vi "Write data to PXImc.vi"(8 "error in (no error)":errorcluster, 11 "RT Data Cluster in":T1 {"StatusRefs" format="%.0x"; "ReceiveRefs"."Data Reference" format="%.0x"; "SendRefs"."Data Reference" format="%.0x"}) -> (0 "error out":errorcluster, 3 "RT Data Cluster out":T1 {"StatusRefs" format="%.0x"; "ReceiveRefs"."Data Reference" format="%.0x"; "SendRefs"."Data Reference" format="%.0x"})   [LabVIEW 2012, in "PXImc Engine.lvlib"]
uses:
  PXImc Engine.lvlib
  RT Data Cluster.ctl
  Shared/Compiled Data.ctl
  <vilib>/NI Veristand/Custom Device API/Block Data Reference.ctl
  <vilib>/NI Veristand/Custom Device API/Data Reference.ctl
  <vilib>/NI Veristand/Custom Device API/Global Data Refs.vi
  <vilib>/pximc/Write (DBL).vi
  <vilib>/pximc/nipximc.lvlib
  <vilib>/NI Veristand/Custom Device API/Custom Device API.lvlib
  <resource>/objmgr/pximc.rc
  Shared/PXImc Shared.lvlib
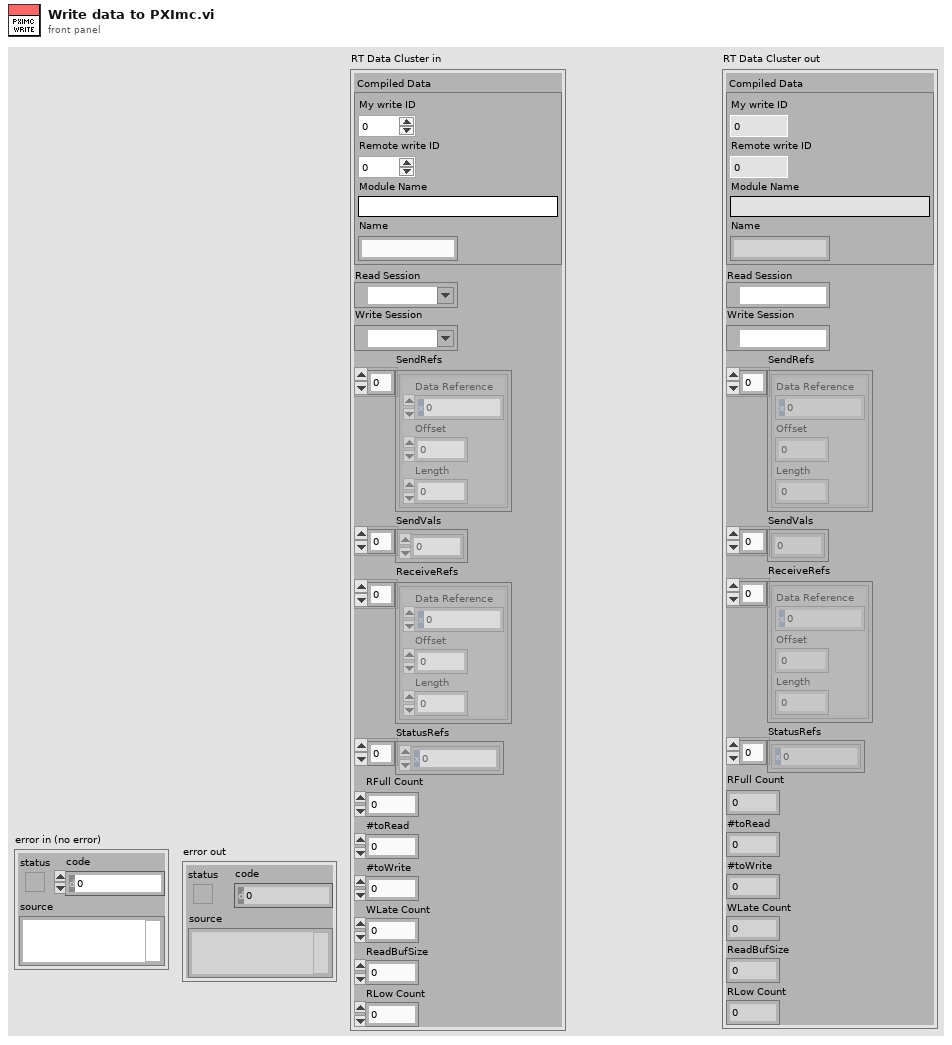
[diagram p1: front panel]
types:
  T1 = typedef "PXImc Engine.lvlib/RT Data Cluster.ctl" = cluster{"Compiled Data":T2, "Read Session":refnum<k21>, "Write Session":refnum<k21>, "SendRefs":T3[], "SendVals":dbl[], "ReceiveRefs":T3[], "StatusRefs":T4[], "RFull Count":dbl, "#toRead":i32, "#toWrite":i32, "WLate Count":dbl, "ReadBufSize":i32, "RLow Count":dbl}
  T2 = typedef "PXImc Shared.lvlib/Compiled Data.ctl" = cluster{"My write ID":u16, "Remote write ID":u16, "Module Name":string, "Name":string}
  T3 = typedef "Custom Device API.lvlib/Block Data Reference.ctl" = cluster{"Data Reference":T4, "Offset":i32, "Length":i32}
  T4 = typedef "Custom Device API.lvlib/Data Reference.ctl" = i32
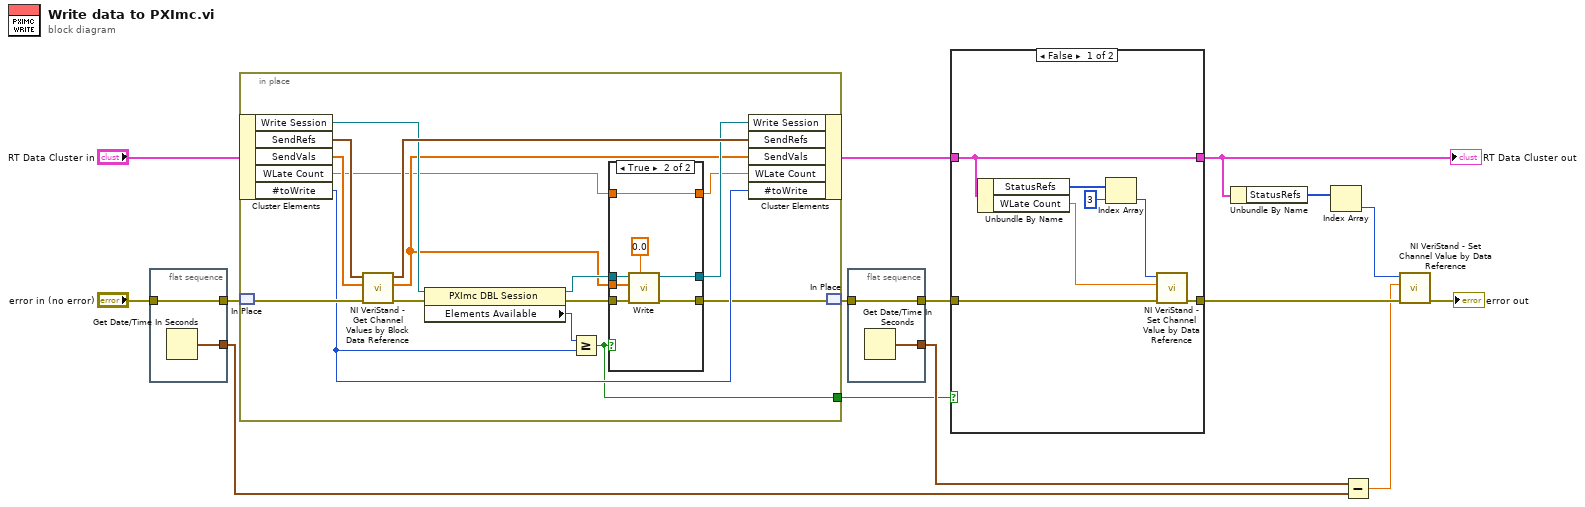
[diagram p0: block diagram]
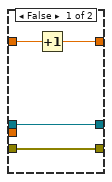
[diagram p3: hidden frame]
diagram:
  n1 = flat-sequence {
    tunnel: [w17] -> w15
    tunnel: "error in (no error)" -> [w17]
    tunnel: [w16] -> w8
    frame #0 {
      n2 = Get Date/Time In Seconds() -> (seconds since 1Jan1904=w16:timestamp)
    }
  }
  n3 = in-place {
    in-place-border: [w18] -> w1
    n4 = in-place-cluster #1("RT Data Cluster in") -> ("Write Session"=w25:refnum<k21>, "SendRefs"=w31:T3[], "SendVals"=w32:dbl[], "WLate Count"=w20:dbl, "#toWrite"=w27:i32)
    n5 = in-place-match #2(w15) -> (w33:errorcluster)
    n6 = call <vilib>:"NI VeriStand - Get Channel Values by Block Data Reference.vi"("error in (no error)"=w33, "Values Array in"=w32, "Block Data Ref"=w31) -> ("error out"=w30:errorcluster, "Values Array out"=w21:dbl[], "Block Data Ref dup"=w29:T3[])  [unwired: 6 in]
    n7 = property class="PXImc DBL Session"(reference=w25, error in=w30) -> (reference out=w24:refnum<k21>, error out=w26:errorcluster, "Elements Available"=w23:u64)
    n8 = Greater Or Equal?(x=w23, y=w27) -> (x >= y?=w18:bool)
    n9 = case shown="True" w18 {
      tunnel: [w35 w44] -> w28
      tunnel: w26 -> [w34 w42]
      tunnel: w24 -> [w35 w41]
      tunnel: [w34 w40] -> w22
      tunnel: w21 -> [_ w39]
      tunnel: w20 -> [w37 w38]
      tunnel: [w36 w38] -> w19
      frame False {
        n10 = Increment(x=w37) -> (x+1=w36:dbl)
      }
      frame True {
        n11 = call-poly <vilib>:"Write.vi"("timeout in seconds (5)"=0.0, "error in (no error)"=w42, "data"=w39, "session in"=w41) -> ("error out"=w40:errorcluster, "session out"=w44:refnum<k21>)  [unwired: 5 in, 1 out]
      }
    }
    n12 = in-place-cluster #1("Write Session"=w28, "SendRefs"=w29, "SendVals"=w21, "WLate Count"=w19, "#toWrite"=w27) -> (w10:T1)
    n13 = in-place-match #2(w22) -> (w12:errorcluster)
  }
  n14 = flat-sequence {
    tunnel: [w46] -> w11
    tunnel: w12 -> [w46]
    tunnel: [w45] -> w9
    frame #0 {
      n15 = Get Date/Time In Seconds() -> (seconds since 1Jan1904=w45:timestamp)
    }
  }
  n16 = case shown="False" w1 {
    tunnel: w11 -> [w53 w55]
    tunnel: w10 -> [w47 w54]
    tunnel: [w48 w55] -> w7
    tunnel: [w47 w54] -> w3
    frame False {
      n17 = Unbundle By Name(w47) -> ("StatusRefs"=w52:T4[], "WLate Count"=w49:dbl)
      n18 = Index Array(array=w52, index=3) -> (element=w50:T4)
      n19 = call <vilib>:"NI VeriStand - Set Channel Value by Data Reference.vi"("error in (no error)"=w53, "Value"=w49, "Data Reference in"=w50) -> ("error out"=w48:errorcluster)  [unwired: 8 in]
    }
    frame True {
    }
  }
  "RT Data Cluster out" <- w3
  n20 = Unbundle By Name(w3) -> ("StatusRefs"=w6:T4[])
  n21 = Index Array(array=w6) -> (element=w5:T4)  [unwired: 1 in]
  n22 = Subtract(x=w9, y=w8) -> (x-y=w4:dbl)
  n23 = call <vilib>:"NI VeriStand - Set Channel Value by Data Reference.vi"("error in (no error)"=w7, "Value"=w4, "Data Reference in"=w5) -> ("error out"=→"error out":errorcluster)  [unwired: 8 in]
